vi "SandBoxAmc.vi"() -> ()   [LabVIEW 2019]
uses:
  MessageAMC_class/MessageAMC.lvclass
  <vilib>/NI/AMC/AMC.lvlib
panel:
  out "error out 2":errorcluster
  out "UDP port used":u16=54321
  out "timed out?":bool
  in  "timeout (25000 ms)":i32=25000
  in  "value":string="VAL"
  in  "name":string="TECT123"
  in  "receiver port (0)":u16=54321
  in  "receiver host":string="192.168.1.10"
  in  "receiver process":string="STAND"
  in  "Send":bool
  in  "stop":bool
  out "error out":errorcluster
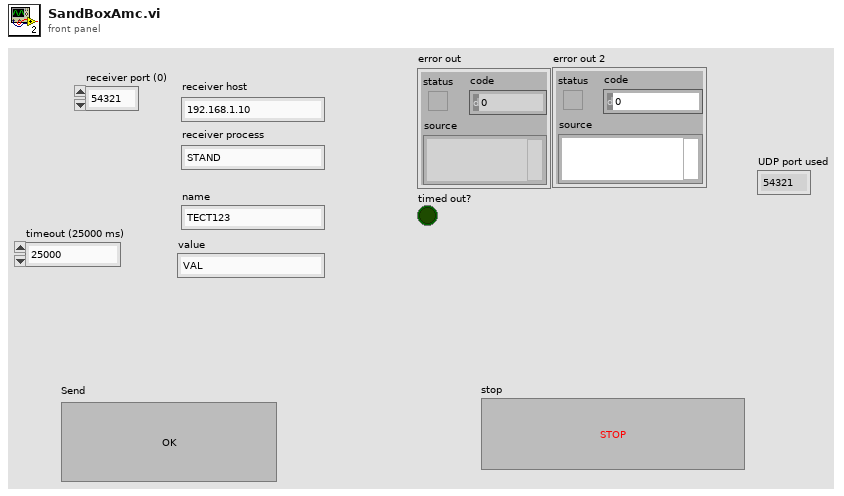
[diagram p1: front panel]
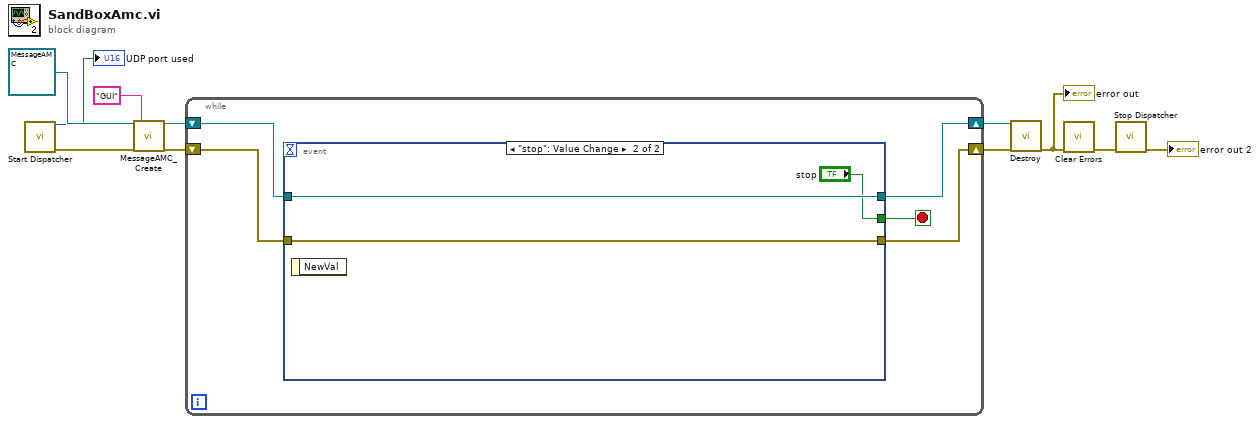
[diagram p0: block diagram]
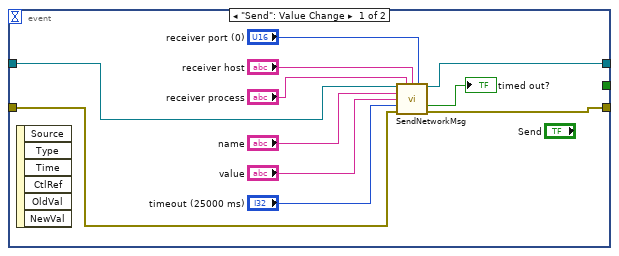
[diagram p2: hidden frame]
diagram:
  n1 = call <vilib>:"Start Dispatcher.vi"() -> ("UDP port used"=→"UDP port used":u16, "error out"=w4:errorcluster)  [unwired: 13 in, 1 out]
  n2 = call "MessageAMC_Create.vi"("reference in"=refnum<class "MessageAMC.lvclass"> refnum, "error in (no error)"=w4, "message queue name"="GUI") -> ("amc"=w9:refnum<class "MessageAMC.lvclass">, "error out"=w8:errorcluster)  [unwired: 15 in]
  n3 = while {
    shift-right: [w14] -> w7
    shift-left: w9 -> [w16]
    shift-right: [w13] -> w6
    shift-left: w8 -> [w15]
    stop <- w12 stop-if-true
    n4 = event shown="[1] \"stop\": Value Change" {
      selector: _ -> [_ _]
      dyn-events: _ -> [_ _]
      timeout: _ -> [_ _]
      tunnel: w16 -> [w27 w30]
      tunnel: w15 -> [w26 w29]
      tunnel: [w25 w30] -> w14
      tunnel: [w24 w29] -> w13
      tunnel: [_ "stop"] -> w12
      event "Send": Value Change {
        n5 = event-data() -> ()  [unwired: 1 in, 6 out]
        n6 = call-dynamic "SendNetworkMsg.vi"("reference in"=w27, "receiver process"="receiver process", "receiver host"="receiver host", "receiver port (0)"="receiver port (0)", "name"="name", "value"="value", "timeout (25000 ms)"="timeout (25000 ms)", "error in (no error)"=w26) -> ("reference out"=w25:refnum<class "MessageAMC.lvclass">, "timed out?"=→"timed out?":bool, "error out"=w24:errorcluster)  [unwired: 5 in]
      }
      event "stop": Value Change {
        n7 = event-data() -> ()  [unwired: 1 in, 1 out]
      }
    }
  }
  n8 = call-dynamic "Destroy.vi"("reference in"=w7, "error in (no error)"=w6) -> ("error out"=w3:errorcluster)  [unwired: 16 in, 1 out]
  "error out" <- w3
  n9 = call <vilib>:"Clear Errors.vi"("error in (no error)"=w3) -> ("error out"=w2:errorcluster)  [unwired: 5 in, 1 out]
  n10 = call <vilib>:"Stop Dispatcher.vi"("error in"=w2) -> ("error out"=→"error out 2":errorcluster)  [unwired: 14 in]
